vi "Actor Core.vi"(8 "error in":errorcluster, 11 "Example View in":refnum<class "Example View.lvclass">) -> (0 "error out":errorcluster, 3 "Actor out":refnum<class "Actor.lvclass">)   [LabVIEW 2023, in "Example MVC Actors.lvlib" / "Example View.lvlib" / "Example View.lvclass"]
doc: "(<B>Filename</B>: Actor Framework.lvlib:Actor.lvclass:Actor Core.vi)\n\nReceives messages to the actor, reacts to them, and initiates any error handling that may shut the actor down.\n\nDescendant classes may override this VI to append parallel tasks for the actor to complete while it handles messages. Overrides use the Call Parent Method node."
uses:
  Example View.lvclass
  C:/Program Files/National Instruments/LabVIEW 2023/vi.lib/ActorFramework/Actor/Actor.lvclass
  C:/Projects/Shared Libraries/Event Actors/View/View.lvclass
  <vilib>/ActorFramework/Actor/Actor.lvclass
  Example View.lvclass/Example View.ctl
  <vilib>/ActorFramework/Actor/Actor.lvclass/Actor.ctl
  <vilib>/ActorFramework/Message Enqueuer/Message Enqueuer.lvclass/Message Enqueuer.ctl
  View/View.lvclass/View.ctl
  Example Events/Boolean Event.lvclass
  C:/Projects/Shared Libraries/Event Actors/Event Data Types/Event Boolean/Event Boolean.lvclass
  C:/Projects/Shared Libraries/Event Actors/Event/Event.lvclass
  Example Events/Double Array Event.lvclass
  Event/Event.lvclass/Event.ctl
  Example View Messages/Update Array Event Msg/Update Array Event Msg.lvclass
  C:/Projects/Shared Libraries/Event Actors/Event Handlers/Abstract Event Message for View/Abstract Event Message for View.lvclass
  Example Events/Timestamp Event.lvclass
  Example View Messages/Update Time Event Msg/Update Time Event Msg.lvclass
  View/properties/Read Name.vi
  <vilib>/ActorFramework/Message Enqueuer/Init from Existing Queue.vi
  <vilib>/ActorFramework/Message Enqueuer/Message Enqueuer.lvclass
  View/View.lvclass
  Event/Event.lvclass
  View Messages/Register Event Msg/Register Event Msg.lvclass
  View Messages/Unregister Event Msg/Unregister Event Msg.lvclass
  View Messages/Generate and Broadcast Event Msg/Generate and Broadcast Event Msg.lvclass
panel:
  in  "Registered for Time":bool=TRUE
  in  "Registered for Data":bool=TRUE
  out "Inited At":string
  out "View Name":string
  in  "Boolean":bool
  out "Time":string
  out "Waveform Graph":dbl[](graph)
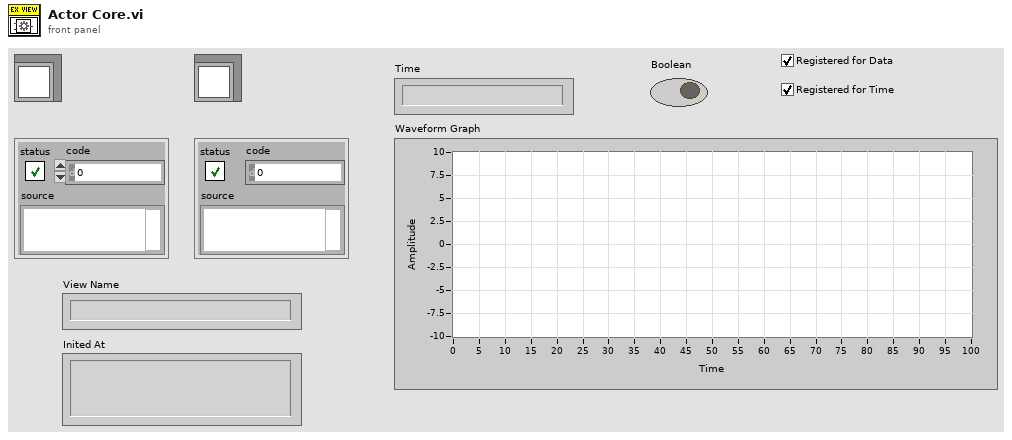
[diagram p1: front panel]
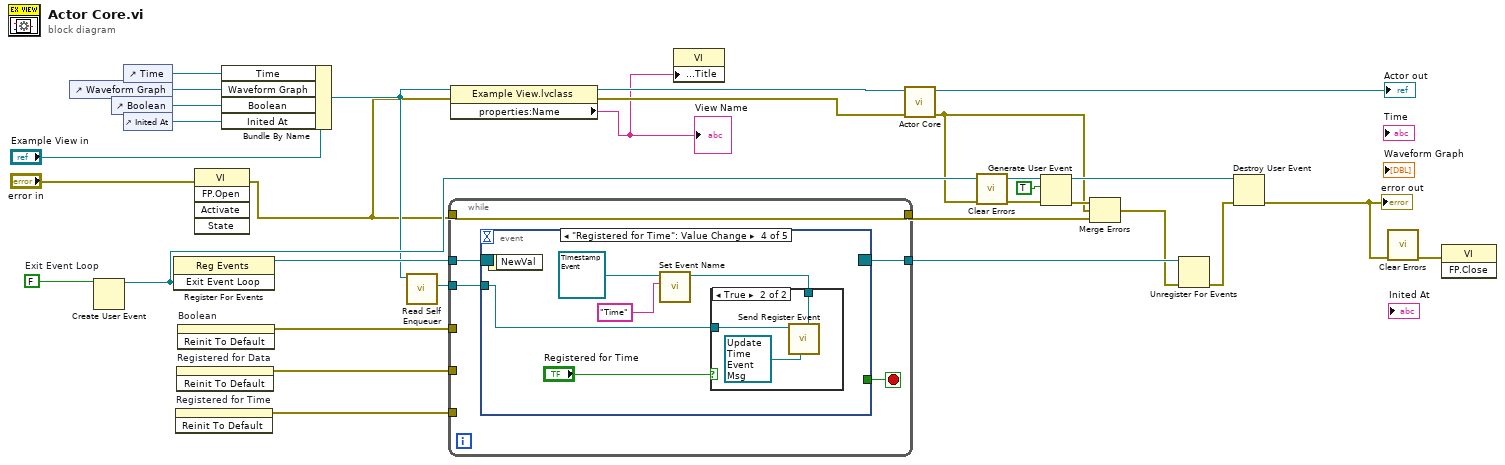
[diagram p0: block diagram]
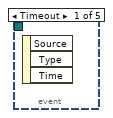
[diagram p2: hidden frame]
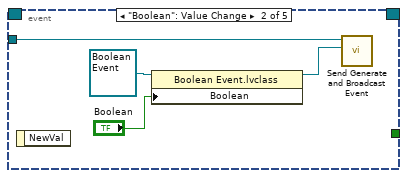
[diagram p3: hidden frame]
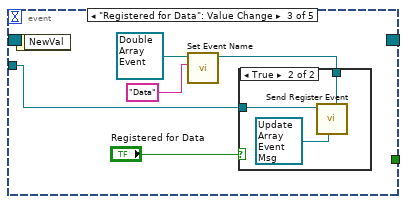
[diagram p4: hidden frame]
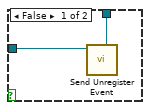
[diagram p5: hidden frame]
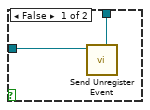
[diagram p6: hidden frame]
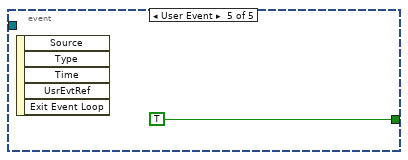
[diagram p7: hidden frame]
diagram:
  w23 = FALSE  # Exit Event Loop
  n1 = control-ref of="Waveform Graph"() -> (w27:refnum<vi>)
  n2 = Create User Event(user event datatype=w23) -> (user event=w20:refnum<user-event>)  [unwired: 1 in, 1 out]
  n3 = control-ref of="Boolean"() -> (w26:refnum<vi>)
  n4 = control-ref of="Time"() -> (w28:refnum<vi>)
  n5 = control-ref of="Inited At"() -> (w4:refnum<vi>)
  n6 = register-events(w20) -> (reference out=w22:refnum<event-registration>)  [unwired: 2 in, 1 out]
  n7 = invoke on="Registered for Time" class="Bool (strict)" method="Reinit To Default"() -> (error out=w1:errorcluster)  [unwired: 3 in, 2 out]
  n8 = invoke on="Registered for Data" class="Bool (strict)" method="Reinit To Default"() -> (error out=w2:errorcluster)  [unwired: 3 in, 2 out]
  n9 = invoke on="Boolean" class="Bool (strict)" method="Reinit To Default"() -> (error out=w3:errorcluster)  [unwired: 3 in, 2 out]
  n10 = invoke class="VI" method="FP.Open"(error in="error in") -> (error out=w7:errorcluster)  [unwired: 4 in, 4 out]
  n11 = Bundle By Name(cluster="Example View in", "Time"=w28, "Waveform Graph"=w27, "Boolean"=w26, "Inited At"=w4) -> (w15:refnum<class "Example View.lvclass">)
  n12 = call <vilib>:"Read Self Enqueuer.vi"("Actor"=w15) -> ("Self Enqueuer"=w24:refnum<class "Message Enqueuer.lvclass">)  [unwired: 10 in]
  n13 = while {
    tunnel: w24 -> [w35]
    tunnel: w22 -> [w34]
    tunnel: w7 -> [w33]
    tunnel: [w33] -> w14
    tunnel: [w32] -> w18
    tunnel: w3 -> [_]
    tunnel: w2 -> [_]
    tunnel: w1 -> [_]
    stop <- w31 stop-if-true
    n14 = event shown="[3] \"Registered for Time\": Value Change" {
      selector: w34 -> [_ _ _ _ _]
      dyn-events: [_ _ _ _ _] -> w32
      timeout: _ -> [_ _ _ _ _]
      tunnel: w35 -> [_ w39 w40 w53 _]
      tunnel: [_ _ _ _ TRUE] -> w31
      event Timeout {
        n15 = event-data() -> ()  [unwired: 1 in, 3 out]
      }
      event "Boolean": Value Change {
        n16 = event-data() -> ()  [unwired: 1 in, 1 out]
        n17 = property class="Boolean Event.lvclass"(reference=refnum<class "Boolean Event.lvclass"> refnum ("Example Source.lvlib:Boolean Event.lvclass"), "Boolean"="Boolean") -> (reference out=w36:refnum<class "Boolean Event.lvclass">)  [unwired: 1 in, 1 out]
        n18 = call "Send Generate and Broadcast Event.vi"("Event Data"=w36, "Message Enqueuer in"=w39) -> ()  [unwired: 8 in, 2 out]
      }
      event "Registered for Data": Value Change {
        n19 = event-data() -> ()  [unwired: 1 in, 1 out]
        n20 = call "Set Event Name.vi"("Name (Generic)"="Data", "Event In"=refnum<class "Double Array Event.lvclass"> refnum ("Double Array Event.lvclass")) -> ("Event Out"=w44:refnum<class "Double Array Event.lvclass">)  [unwired: 9 in]
        n21 = case shown="True" "Registered for Data" {
          tunnel: w44 -> [w46 w49]
          tunnel: w40 -> [w45 w47]
          frame False {
            n22 = call "Send Unregister Event.vi"("Event"=w46, "Message Enqueuer in"=w45) -> ()  [unwired: 8 in, 2 out]
          }
          frame True {
            n23 = call "Send Register Event.vi"("Event"=w49, "Event Handler"=refnum<class "Update Array Event Msg.lvclass"> refnum ("Update Array Msg.lvclass"), "Message Enqueuer in"=w47) -> ()  [unwired: 7 in, 2 out]
          }
        }
      }
      event "Registered for Time": Value Change {
        n24 = event-data() -> ()  [unwired: 1 in, 1 out]
        n25 = call "Set Event Name.vi"("Name (Generic)"="Time", "Event In"=refnum<class "Timestamp Event.lvclass"> refnum ("Timestamp Event.lvclass")) -> ("Event Out"=w54:refnum<class "Timestamp Event.lvclass">)  [unwired: 9 in]
        n26 = case shown="True" "Registered for Time" {
          tunnel: w54 -> [w56 w59]
          tunnel: w53 -> [w55 w58]
          frame False {
            n27 = call "Send Unregister Event.vi"("Event"=w56, "Message Enqueuer in"=w55) -> ()  [unwired: 8 in, 2 out]
          }
          frame True {
            n28 = call "Send Register Event.vi"("Event"=w59, "Event Handler"=refnum<class "Update Time Event Msg.lvclass"> refnum ("Update Time Msg.lvclass"), "Message Enqueuer in"=w58) -> ()  [unwired: 7 in, 2 out]
          }
        }
      }
      event User Event {
        n29 = event-data() -> ()  [unwired: 1 in, 5 out]
      }
    }
  }
  n30 = property class="Example View.lvclass"(reference=w15, error in=w7) -> (reference out=w8:refnum<class "Example View.lvclass">, error out=w6:errorcluster, "properties:Name"=w5:string)
  "View Name" <- w5
  n31 = property class="VI"("Front Panel.Title"=w5) -> ()  [unwired: 2 in, 2 out]
  n32 = call-parent "Actor Core.vi"("error in"=w6, "Actor in"=w8) -> ("error out"=w10:errorcluster, "Actor out"=→"Actor out":refnum<class "Actor.lvclass">)  [unwired: 8 in]
  n33 = call <vilib>:"Clear Errors.vi"("error in (no error)"=w10) -> ("error out"=w9:errorcluster)  [unwired: 5 in, 1 out]
  n34 = Generate User Event(user event=w20, event data cluster=TRUE ("event data"), error in=w9) -> (user event out=w19:refnum<user-event>, error out=w21:errorcluster)  [unwired: 1 in]
  n35 = Merge Errors(w21, w10, w14) -> (w11:errorcluster)
  n36 = Unregister For Events(event registration refnum=w18, error in=w11) -> (error out=w17:errorcluster)
  n37 = Destroy User Event(user event=w19, error in=w17) -> (error out=w12:errorcluster)
  "error out" <- w12
  n38 = call <vilib>:"Clear Errors.vi"("error in (no error)"=w12) -> ("error out"=w13:errorcluster)  [unwired: 5 in, 1 out]
  n39 = invoke class="VI" method="FP.Close"(error in=w13) -> ()  [unwired: 2 in, 3 out]
